vi "convertFESTOfromBytes.vi"(9 "Start Byte":i32, 11 "Bytes":u8[](array[numeric])) -> (3 "data":bool[](array[boolean]))   [LabVIEW 2011]
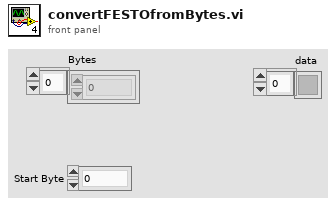
[diagram p1: front panel]
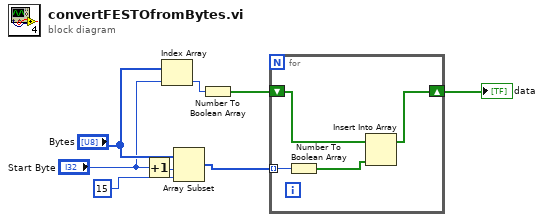
[diagram p0: block diagram]
diagram:
  n1 = Increment(x="Start Byte") -> (x+1=w2:i32)
  n2 = Index Array(array="Bytes", index="Start Byte") -> (element=w6:u8)
  n3 = Array Subset(array="Bytes", index=w2, length=15) -> (w8:u8[])
  n4 = Number To Boolean Array(number=w6) -> (Boolean array=w5:bool[])
  n5 = for {
    tunnel: w8 -> [w12] mode=indexing
    shift-right: [w10] -> w4
    shift-left: w5 -> [w11]
    n6 = Number To Boolean Array(number=w12) -> (Boolean array=w9:bool[])
    n7 = Insert Into Array(array=w11, new element=w9) -> (w10:bool[])  [unwired: 1 in]
  }
  "data" <- w4
